vi "AD2_SDK_Init.vi"(0 "object in":refnum<class "AD2_SDK.lvclass">, 5 "error in (no error)":errorcluster) -> (14 "object out":refnum<class "AD2_SDK.lvclass">, 19 "error out":errorcluster)   [LabVIEW 2019, in "AD2_SDK.lvclass"]
uses:
  AD2_SDK.lvclass
  C:/GIT/ThermalAcousticProject/InstrumentBase_class/AD2_SDK_class/InstrumentBase.lvclass
  AD2_MSO_SDK_class/AD2_MSO_SDK.lvclass
  AD2_WFG_SDK_class/AD2_WFG_SDK.lvclass
  AD2_SDK.lvclass/AD2_SDK.ctl
  InstrumentBase_class/AD2_SDK_class/InstrumentBase.lvclass
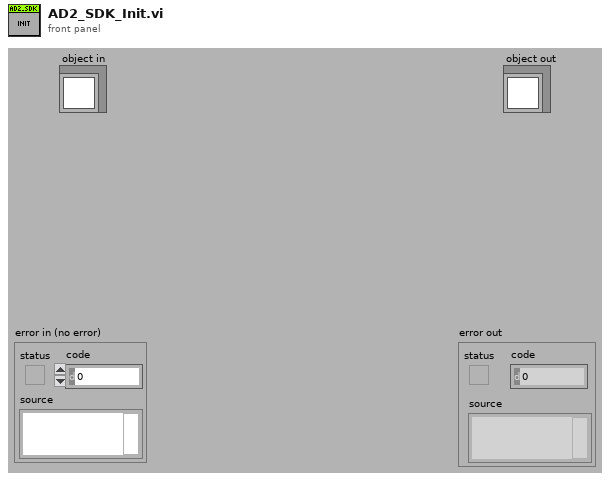
[diagram p1: front panel]
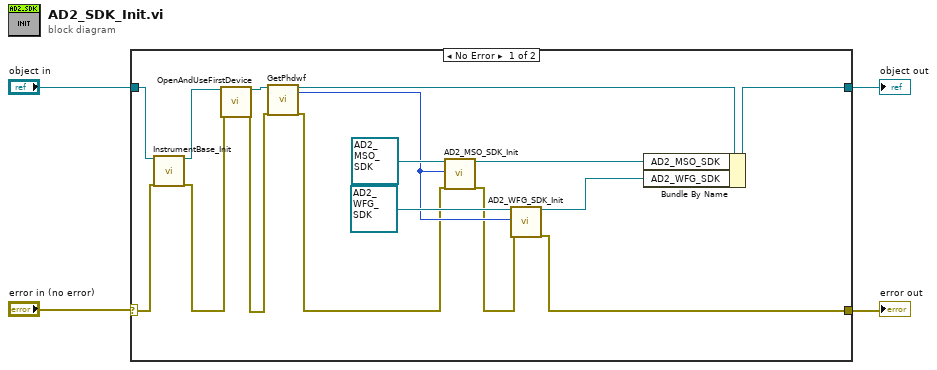
[diagram p0: block diagram]
diagram:
  n1 = case shown="No Error" "error in (no error)" {
    selector: "error in (no error)" -> [w6 w21]
    tunnel: "object in" -> [w8 w22]
    tunnel: [w20 w22] -> w3
    tunnel: [w9 w21] -> w1
    frame No Error {
      n2 = call "InstrumentBase_Init.vi"("object in"=w8, "error in (no error)"=w6) -> ("object out"=w7:refnum<class "AD2_SDK.lvclass">, "error out"=w5:errorcluster)  [unwired: 16 in]
      n3 = call-dynamic "OpenAndUseFirstDevice.vi"("object in"=w7, "error in (no error)"=w5) -> ("object out"=w17:refnum<class "AD2_SDK.lvclass">, "error out"=w16:errorcluster)  [unwired: 16 in]
      n4 = call-dynamic "GetPhdwf.vi"("object in"=w17, "error in (no error)"=w16) -> ("object out"=w10:refnum<class "AD2_SDK.lvclass">, "phdwf"=w13:i32, "error out"=w11:errorcluster)  [unwired: 15 in]
      n5 = call "AD2_MSO_SDK_Init.vi"("object in"=refnum<class "AD2_MSO_SDK.lvclass"> refnum ("AD2_MSO_SDK"), "phdwf"=w13, "error in (no error)"=w11) -> ("object out"=w14:refnum<class "AD2_MSO_SDK.lvclass">, "error out"=w12:errorcluster)  [unwired: 15 in]
      n6 = call "AD2_WFG_SDK_Init.vi"("object in"=refnum<class "AD2_WFG_SDK.lvclass"> refnum ("AD2_SDK"), "phdwf"=w13, "error in (no error)"=w12) -> ("object out"=w18:refnum<class "AD2_WFG_SDK.lvclass">, "error out"=w9:errorcluster)  [unwired: 15 in]
      n7 = Bundle By Name(cluster=w10, "AD2_MSO_SDK"=w14, "AD2_WFG_SDK"=w18) -> (w20:refnum<class "AD2_SDK.lvclass">)
    }
    frame Error {
    }
  }
  "object out" <- w3
  "error out" <- w1
